vi "lOOK AT R140.vi"() -> ()   [LabVIEW 2020]
uses:
  file handler/VFH-VNA_File_Handler.lvlib
panel:
  in  "Stop":bool
  in  "Folder Path":path=path "C:/NanoVNA-App/Recordings/2024-07-26 09-29-22"
  in  "Tab Control":enum32{"Page 1", "Page 2"}(tab)
  out "Complex":cluster{"Frequency":dbl[], "S21_Imag":dbl[]}[](graph)
  in  "Log Raw":bool
  out "Calc":cluster{"Frequency":dbl[], "S11_Imag":dbl[]}[](graph)
  out "Raw":cluster{"Frequency":dbl[], "S21_Imag":dbl[]}[](graph)
  in  "Log calc":bool
  in  "Log complex":bool
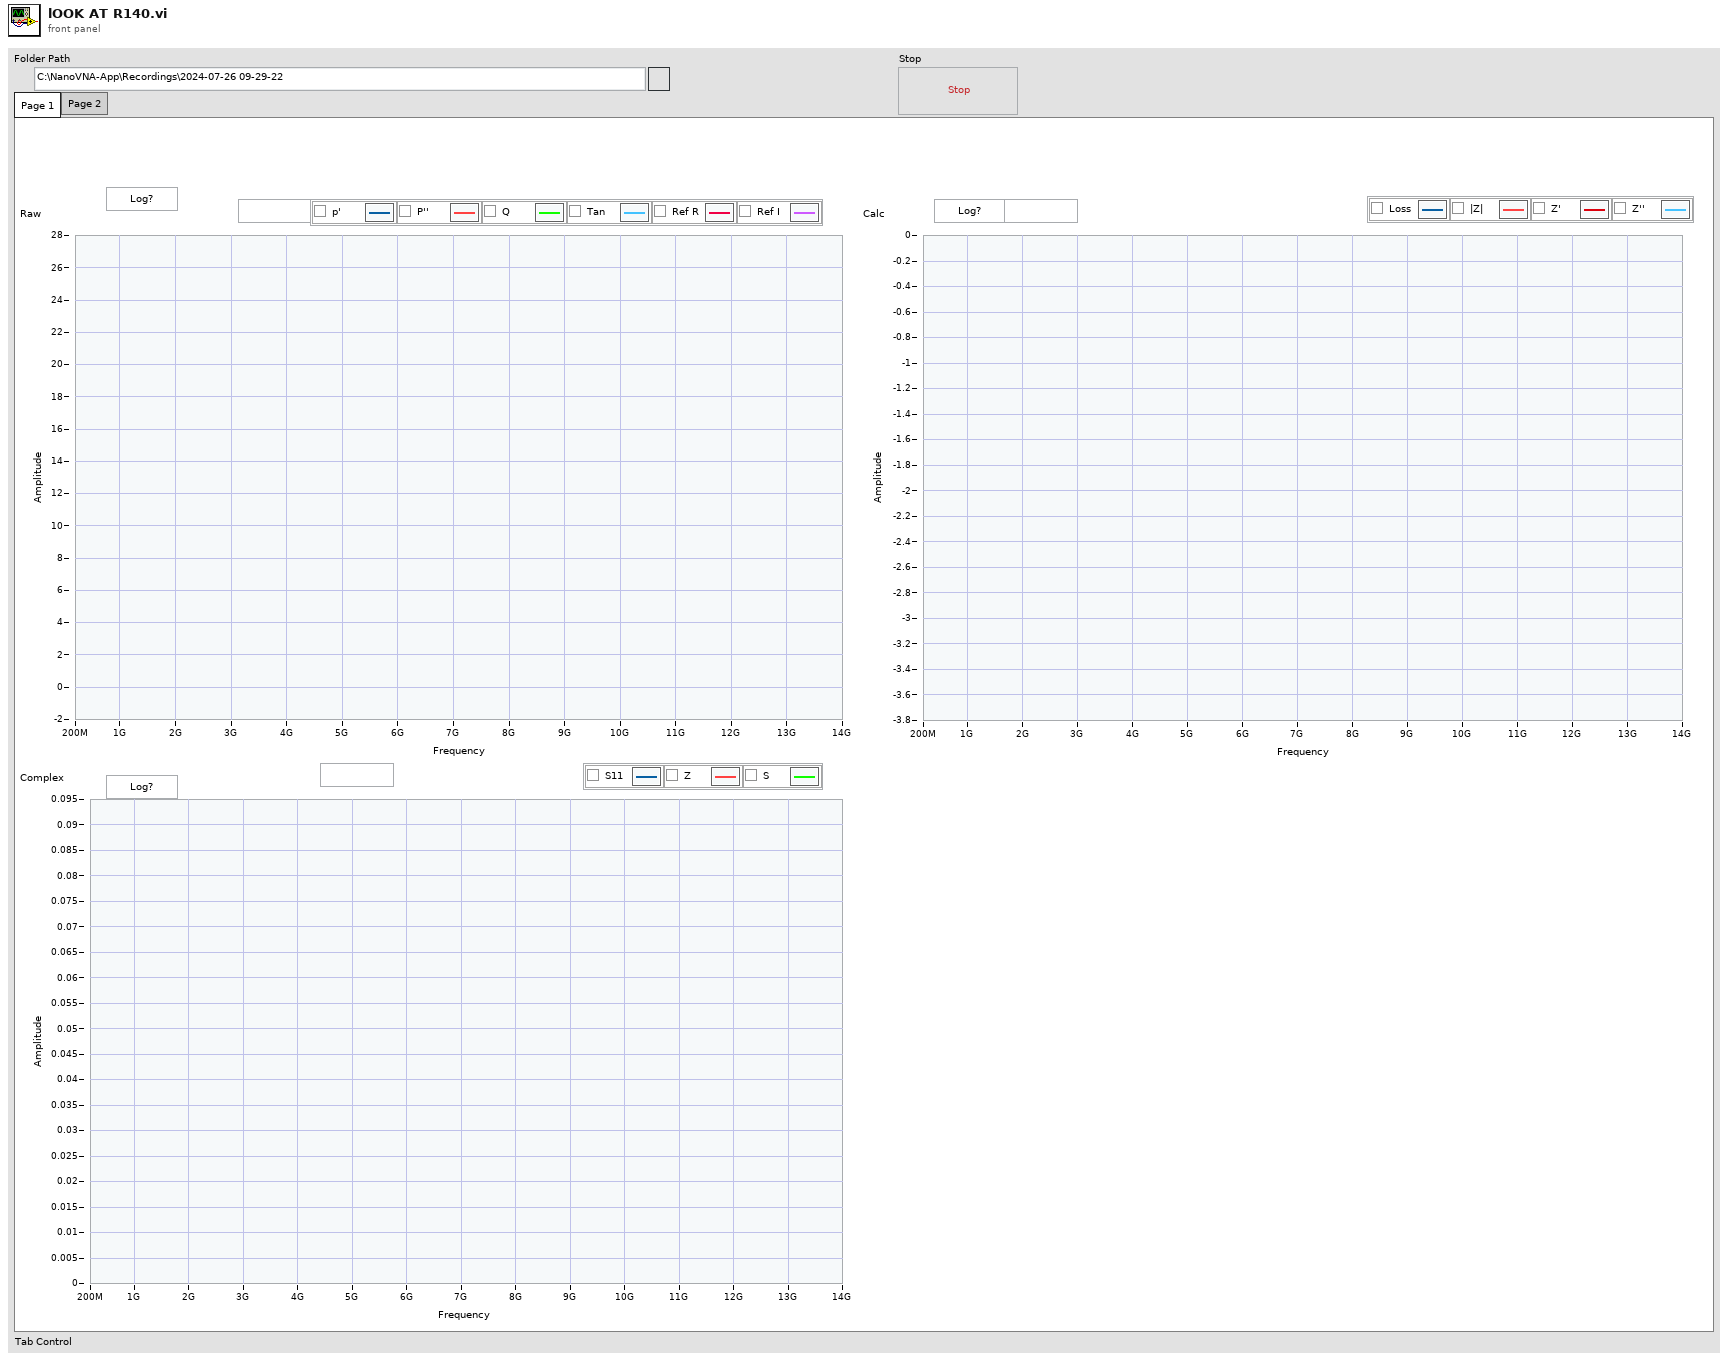
[diagram p1: front panel]
types:
  T1 = typedef "VFH-VNA_File_Handler.lvlib/VFH-file_cluster-Expensive.ctl" = cluster{"Frequency":dbl[], "Permativity'":dbl[], "Permativity''":dbl[], "Q [S/m]":dbl[], "Tan":dbl[], "Reflection R":dbl[], "Reflection I":dbl[]}
  T2 = cluster{"Complex Input":cluster{"Frequency":dbl[], "Array":cdb[]}, "Complex Z":cluster{"Frequency":dbl[], "Array":cdb[]}, "Complex S":cluster{"Frequency":dbl[], "Array":cdb[]}}
  T3 = cluster{"Loss":cluster{"Frequency":dbl[], "Array":dbl[]}, "Z Modulus":cluster{"Frequency":dbl[], "Array":dbl[]}, "Z'":cluster{"Frequency":dbl[], "Array":dbl[]}, "Z''":cluster{"Frequency":dbl[], "Array":dbl[]}}
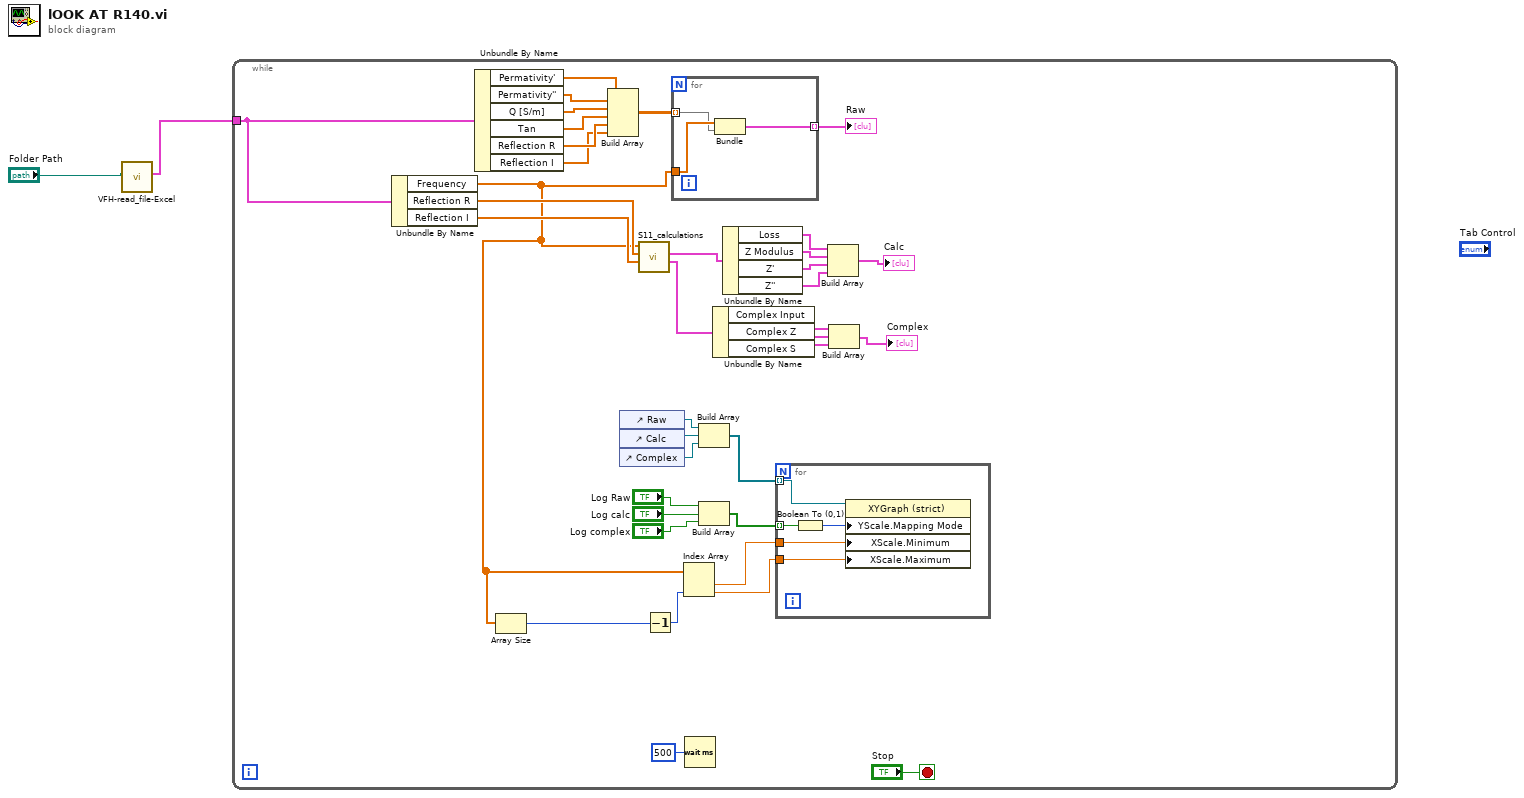
[diagram p0: block diagram]
diagram:
  n1 = call "VFH-read_file-Excel.vi"("file path (dialog if empty)"="Folder Path") -> ("output cluster"=w1:T1)  [unwired: 9 in, 1 out]
  n2 = while {
    tunnel: w1 -> [w3]
    stop <- "Stop" stop-if-true
    n3 = Unbundle By Name(w3) -> ("Frequency"=w5:dbl[], "Reflection R"=w14:dbl[], "Reflection I"=w13:dbl[])
    n4 = Unbundle By Name(w3) -> ("Permativity'"=w12:dbl[], "Permativity''"=w11:dbl[], "Q [S/m]"=w10:dbl[], "Tan"=w9:dbl[], "Reflection R"=w8:dbl[], "Reflection I"=w7:dbl[])
    n5 = Array Size(array=w5) -> (size(s)=w17:i32)
    n6 = Build Array(w12, w11, w10, w9, w8, w7) -> (w6:dbl[][])
    n7 = control-ref of="Raw"() -> (w26:refnum<vi>)
    n8 = control-ref of="Calc"() -> (w25:refnum<vi>)
    n9 = control-ref of="Complex"() -> (w24:refnum<vi>)
    n10 = call "S11_calculations.vi"("S11_Imag"=w13, "S11_Real"=w14, "Frequency"=w5) -> ("Complex"=w29:T2, "Calc"=w39:T3)  [unwired: 6 in, 1 out]
    n11 = Decrement(x=w17) -> (x-1=w16:i32)
    n12 = for {
      tunnel: w6 -> [w41] mode=indexing
      tunnel: w5 -> [w42]
      tunnel: [w40] -> w4 mode=indexing
      n13 = Bundle("Frequency"=w42, w41) -> (w40:cluster{"Frequency":dbl[], dbl[]})  [unwired: 1 in]
    }
    "Raw" <- w4
    n14 = Index Array(array=w5, index #2=w16) -> (element #1=w18:dbl, element #2=w15:dbl)  [unwired: 1 in]
    n15 = Wait (ms)(milliseconds to wait=u32 500) -> ()  [unwired: 1 out]
    n16 = Build Array(w26, w25, w24) -> (w23:refnum<vi>[])
    n17 = Build Array("Log Raw", "Log calc", "Log complex") -> (w19:bool[])
    n18 = Unbundle By Name(w29) -> ("Complex Input"=w30:cluster{"Frequency":dbl[], "Array":cdb[]}, "Complex Z"=w31:cluster{"Frequency":dbl[], "Array":cdb[]}, "Complex S"=w32:cluster{"Frequency":dbl[], "Array":cdb[]})
    n19 = Unbundle By Name(w39) -> ("Loss"=w38:cluster{"Frequency":dbl[], "Array":dbl[]}, "Z Modulus"=w37:cluster{"Frequency":dbl[], "Array":dbl[]}, "Z'"=w36:cluster{"Frequency":dbl[], "Array":dbl[]}, "Z''"=w35:cluster{"Frequency":dbl[], "Array":dbl[]})
    n20 = for {
      tunnel: w23 -> [w47] mode=indexing
      tunnel: w19 -> [w46] mode=indexing
      tunnel: w18 -> [w44]
      tunnel: w15 -> [w43]
      n21 = Boolean To (0,1)(Boolean=w46) -> (0, 1=w45:i16)
      n22 = property class="XYGraph (strict)"(reference=w47, "YScale.Mapping Mode"=w45, "XScale.Minimum"=w44, "XScale.Maximum"=w43) -> ()  [unwired: 1 in, 2 out]
    }
    n23 = Build Array(w38, w37, w36, w35) -> (→"Calc":cluster{"Frequency":dbl[], "Array":dbl[]}[])
    n24 = Build Array(w30, w31, w32) -> (→"Complex":cluster{"Frequency":dbl[], "Array":cdb[]}[])
  }
